vi "Get Segmented Log Ref.vi"(8 "error in (no error)":errorcluster, 11 "Triggered Log in":refnum<class "Triggered Log.lvclass">) -> (0 "error out":errorcluster, 2 "Segmented Log Ref":refnum<data-value>, 3 "Triggered Log out":refnum<class "Triggered Log.lvclass">)   [LabVIEW 2015, in "Triggered Log.lvclass"]
uses:
  Triggered Log.lvclass
  Engine/Classes/Logs/Segmented Logs/Segmented Log/Segmented Log.lvclass
  Triggered Log.lvclass/Triggered Log.ctl
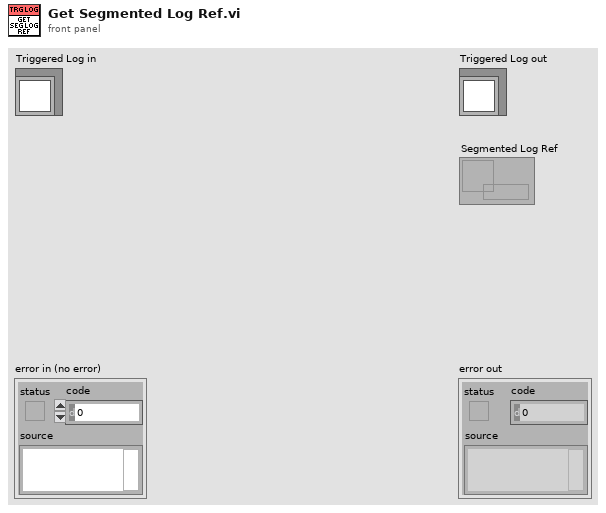
[diagram p1: front panel]
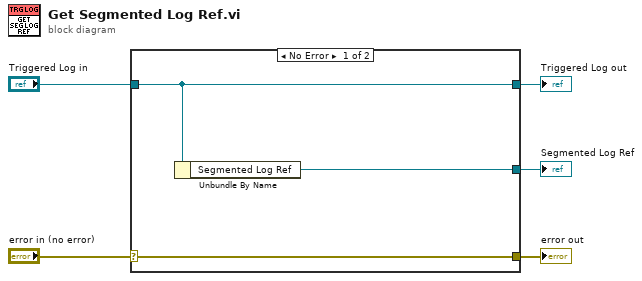
[diagram p0: block diagram]
diagram:
  n1 = case shown="No Error" "error in (no error)" {
    selector: "error in (no error)" -> [w8 w9]
    tunnel: [w8 w9] -> w4
    tunnel: [w7 w10] -> w2
    tunnel: "Triggered Log in" -> [w7 w10]
    tunnel: [w6 _] -> w1
    frame No Error {
      n2 = Unbundle By Name(w7) -> ("Segmented Log Ref"=w6:refnum<data-value>)
    }
    frame Error {
    }
  }
  "error out" <- w4
  "Triggered Log out" <- w2
  "Segmented Log Ref" <- w1
